vi "write_attributes.vi"(8 "error in (no error)":errorcluster caption="entrée d'erreur (pas d'erreur)", 10 "attributes":T1, 11 "Isomap en entrée":refnum<class "Isomap.lvclass">) -> (0 "error out":errorcluster caption="sortie d'erreur", 3 "Isomap en sortie":refnum<class "Isomap.lvclass">)   [LabVIEW 2020, in "Isomap.lvclass"]
uses:
  Isomap.lvclass
  Controls/isomap_attributes.ctl
  Isomap.lvclass/Isomap.ctl
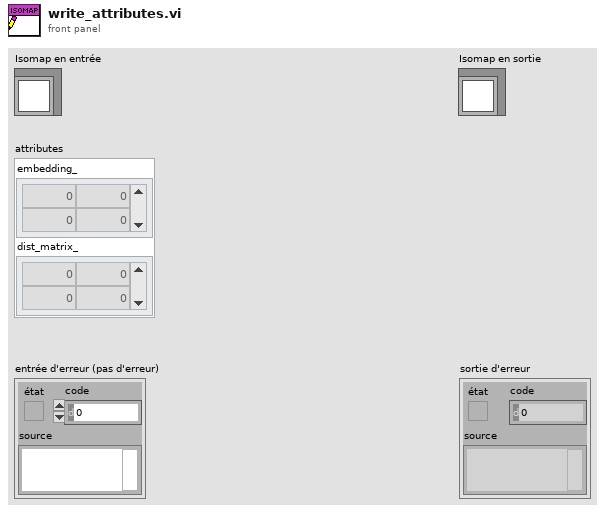
[diagram p1: front panel]
types:
  T1 = typedef "isomap_attributes.ctl" = cluster{"embedding_":dbl[][], "dist_matrix_":dbl[][]}
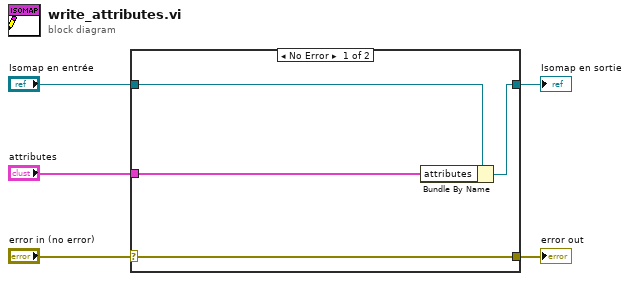
[diagram p0: block diagram]
diagram:
  n1 = case shown="No Error" "error in (no error)" {
    selector: "error in (no error)" -> [w9 w10]
    tunnel: [w9 w10] -> w4
    tunnel: [w7 w11] -> w2
    tunnel: "Isomap en entrée" -> [w8 w11]
    tunnel: "attributes" -> [w6 _]
    frame No Error {
      n2 = Bundle By Name(cluster=w8, "attributes"=w6) -> (w7:refnum<class "Isomap.lvclass">)
    }
    frame Error {
    }
  }
  "error out" <- w4
  "Isomap en sortie" <- w2
